vi "Get ROI X-Y.vi"(11 "Base Graph in":refnum<class "Base Graph.lvclass">) -> (2 "ROI XY":T1, 3 "Base Graph out":refnum<class "Base Graph.lvclass">)   [LabVIEW 2023, in "Base Graph.lvclass"]
uses:
  Base Graph.lvclass
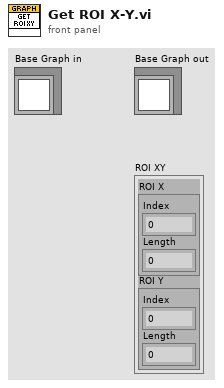
[diagram p1: front panel]
types:
  T1 = cluster{"ROI X":cluster{"Index":u32, "Length":u32}, "ROI Y":cluster{"Index":u32, "Length":u32}}
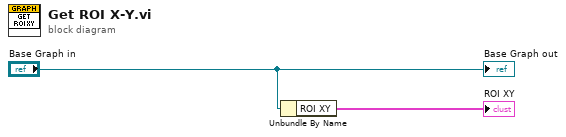
[diagram p0: block diagram]
diagram:
  n1 = Unbundle By Name("Base Graph in") -> ("ROI XY"=→"ROI XY":T1)
  "Base Graph out" <- "Base Graph in"
